vi "CubSolder.vi"() -> ()   [LabVIEW 2019]
panel:
  out "error out 2":errorcluster
  out "read string 8":string
  out "read string 7":string
  out "read string 6":string
  out "read string 5":string
  out "read string 4":string
  out "read string 3":string
  out "read string 2":string
  out "hex integer string":string
  in  "String":string="\\9F\\9F\\95\\99\\9D\\E5\\9F\\9F\\99\\8F\\A7"
  out "error out":errorcluster
  out "read string":string
  # "5C39 465C"
  # "\\9F\\9F\\97\\9F\\A7\\9F\\9F\\95\\99\\99\\E5"
  # "?      02FE"
  # "1A"
  # "9F 9F 97 9F"
  # "BFEA F98D 9B"
  # "BFEA F98D 9B"
  # "3246"
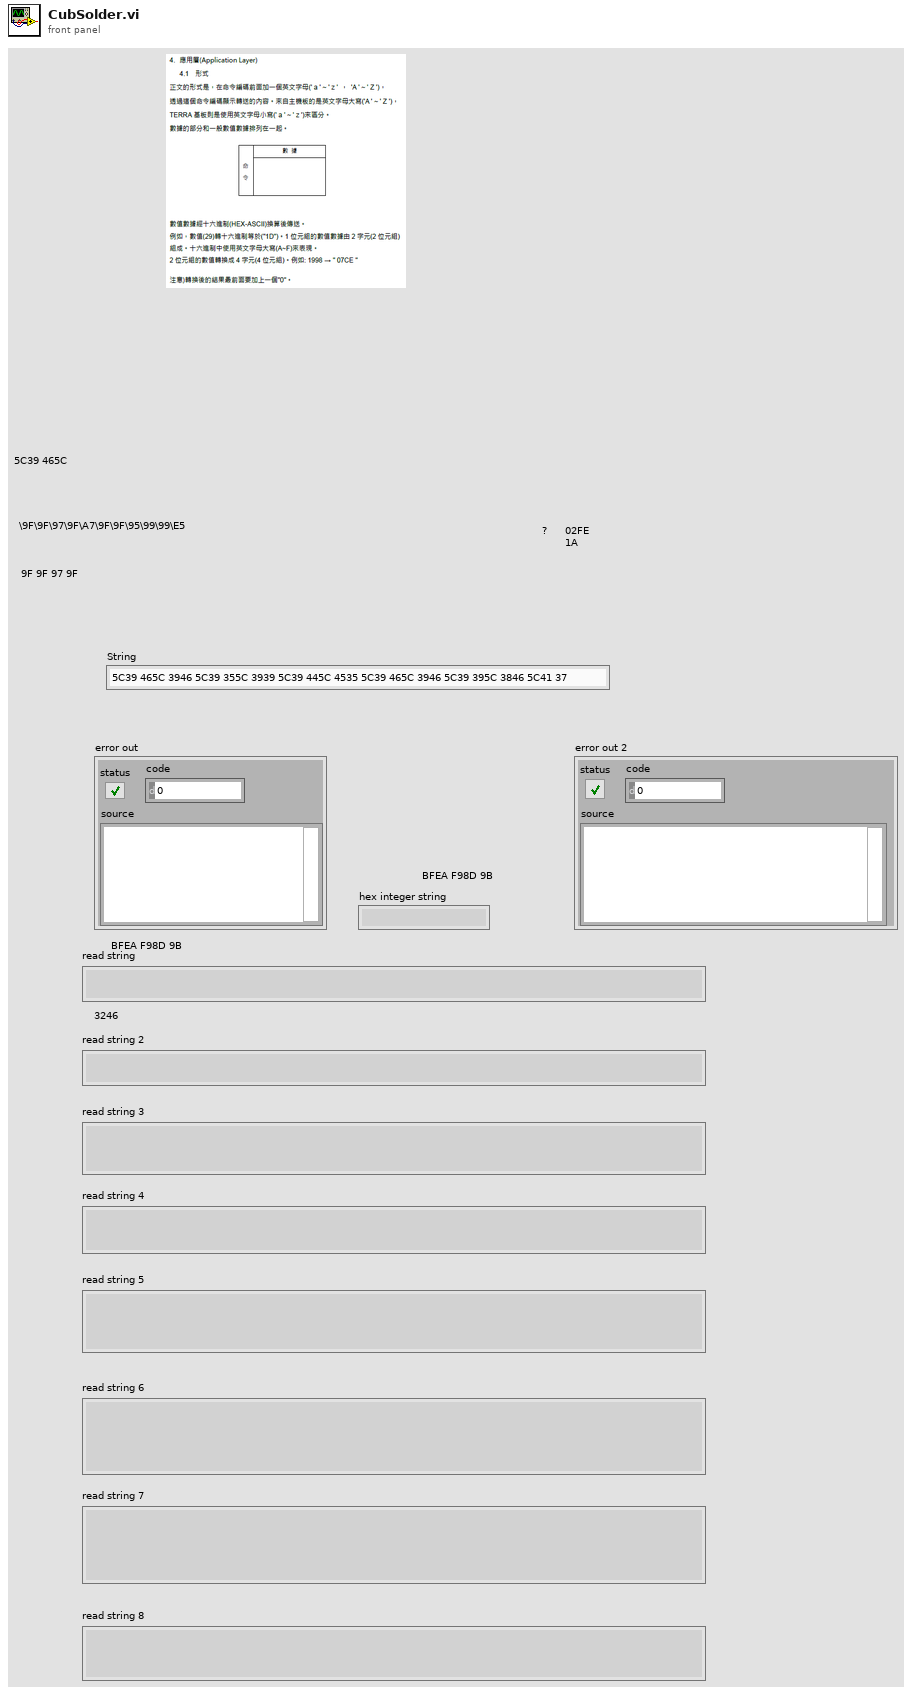
[diagram p1: front panel]
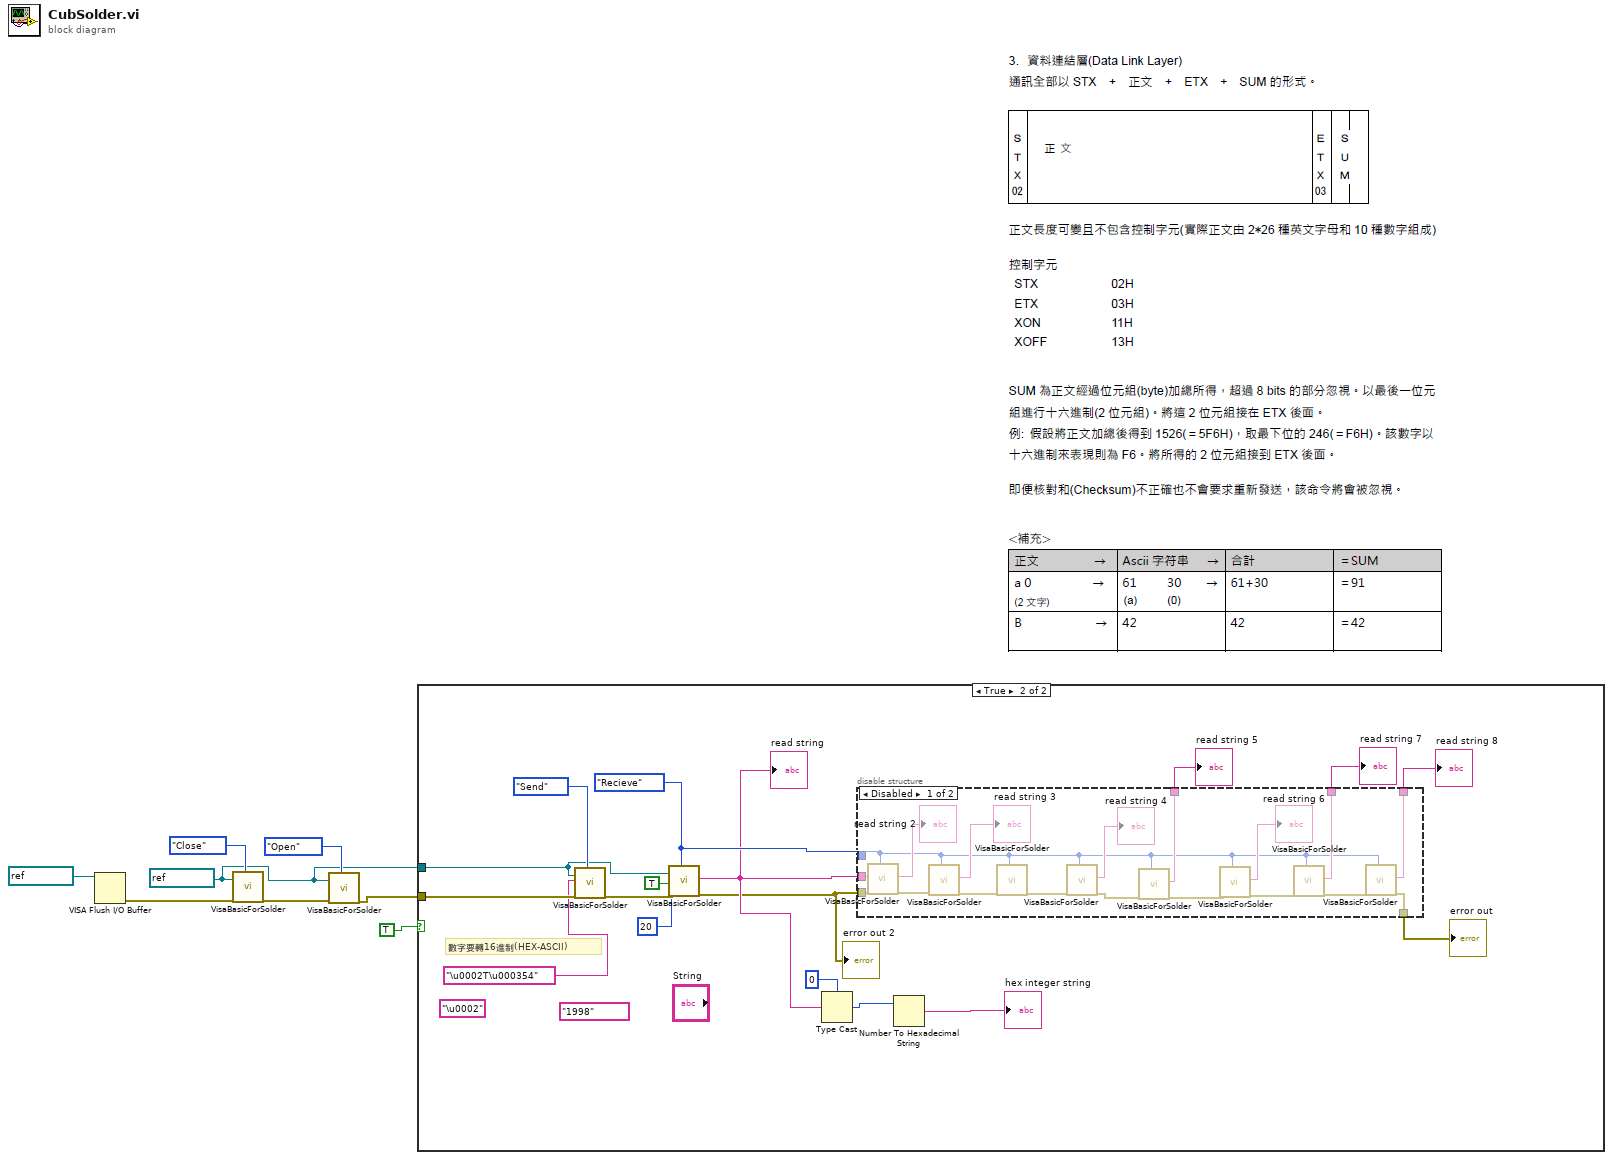
[diagram p0: block diagram]
diagram:
  w3 = refnum<visa-resource-name> "COM3" ("VISA resource name")
  n1 = VISA Flush I/O Buffer(VISA resource name=refnum<visa-resource-name> "COM3") -> (error out=w1:errorcluster)  [unwired: 2 in, 1 out]
  n2 = call "VisaBasicForSolder.vi"("VISA resource name"=w3, "error in (no error)"=w1, "VisaAction"=enum16{"Open", "Send", "Recieve", "Close"}."Close") -> ("error out"=w6:errorcluster)  [unwired: 15 in, 1 out]
  n3 = call "VisaBasicForSolder.vi"("VISA resource name"=w3, "error in (no error)"=w6, "VisaAction"=enum16{"Open", "Send", "Recieve", "Close"}."Open") -> ("error out"=w4:errorcluster)  [unwired: 15 in, 1 out]
  n4 = case shown="True" TRUE {
    tunnel: w4 -> [_ w24]
    tunnel: w3 -> [_ w21]
    frame False {
    }
    frame True {
      w13 = enum16{"Open", "Send", "Recieve", "Close"}."Recieve" ("VisaAction")
      (unwired) "1998"
      (unwired) "\u0002"
      # "數字要轉16進制(HEX-ASCII)"
      n5 = call "VisaBasicForSolder.vi"("VISA resource name"=w21, "Cmd"="\u0002T\u000354", "error in (no error)"=w24, "VisaAction"=enum16{"Open", "Send", "Recieve", "Close"}."Send") -> ("error out"=w22:errorcluster)  [unwired: 14 in, 1 out]
      n6 = call "VisaBasicForSolder.vi"("VISA resource name"=w21, "TimeOut"=TRUE, "Time(0.1)"=u32 20, "error in (no error)"=w22, "VisaAction"=w13) -> ("read string"=w10:string, "error out"=w9:errorcluster)  [unwired: 13 in]
      "read string" <- w10
      "error out 2" <- w9
      n7 = Type Cast(type=0, x=w10) -> (*(type *) &x=w19:i32)
      n8 = disable-structure shown="Disabled" {
        disable-tunnel: [w40 _] -> w15
        disable-tunnel: [w38 _] -> w14
        disable-tunnel: w13 -> [w37 _]
        disable-tunnel: [w36 _] -> w12
        disable-tunnel: [w35 _] -> w11
        disable-tunnel: w10 -> [w34 _]
        disable-tunnel: w9 -> [w33 _]
        frame Disabled {
          n9 = call "VisaBasicForSolder.vi"("Cmd"=w34, "error in (no error)"=w33, "VisaAction"=w37) -> ("read string"=→"read string 2":string, "error out"=w32:errorcluster)  [unwired: 15 in]
          n10 = call "VisaBasicForSolder.vi"("error in (no error)"=w32, "VisaAction"=w37) -> ("read string"=→"read string 3":string, "error out"=w31:errorcluster)  [unwired: 16 in]
          n11 = call "VisaBasicForSolder.vi"("error in (no error)"=w31, "VisaAction"=w37) -> ("error out"=w30:errorcluster)  [unwired: 16 in, 1 out]
          n12 = call "VisaBasicForSolder.vi"("error in (no error)"=w30, "VisaAction"=w37) -> ("read string"=→"read string 4":string, "error out"=w29:errorcluster)  [unwired: 16 in]
          n13 = call "VisaBasicForSolder.vi"("error in (no error)"=w29, "VisaAction"=w37) -> ("read string"=w40:string, "error out"=w28:errorcluster)  [unwired: 16 in]
          n14 = call "VisaBasicForSolder.vi"("error in (no error)"=w28, "VisaAction"=w37) -> ("read string"=→"read string 6":string, "error out"=w27:errorcluster)  [unwired: 16 in]
          n15 = call "VisaBasicForSolder.vi"("error in (no error)"=w27, "VisaAction"=w37) -> ("read string"=w38:string, "error out"=w26:errorcluster)  [unwired: 16 in]
          n16 = call "VisaBasicForSolder.vi"("error in (no error)"=w26, "VisaAction"=w37) -> ("read string"=w36:string, "error out"=w35:errorcluster)  [unwired: 16 in]
        }
        frame Enabled {
        }
      }
      "error out" <- w11
      "read string 5" <- w15
      "read string 7" <- w14
      "read string 8" <- w12
      n17 = Number To Hexadecimal String(2:w19) -> (0:→"hex integer string":string)  [unwired: 1 in]
    }
  }
